vi "FolderSyncTool.vi"() -> ()   [LabVIEW 2023]
panel:
  out "Log":string
  out "file in tmp dir":path
  out "Copy Complete":bool
  in  "Dest Path":path
  in  "Source Path":path
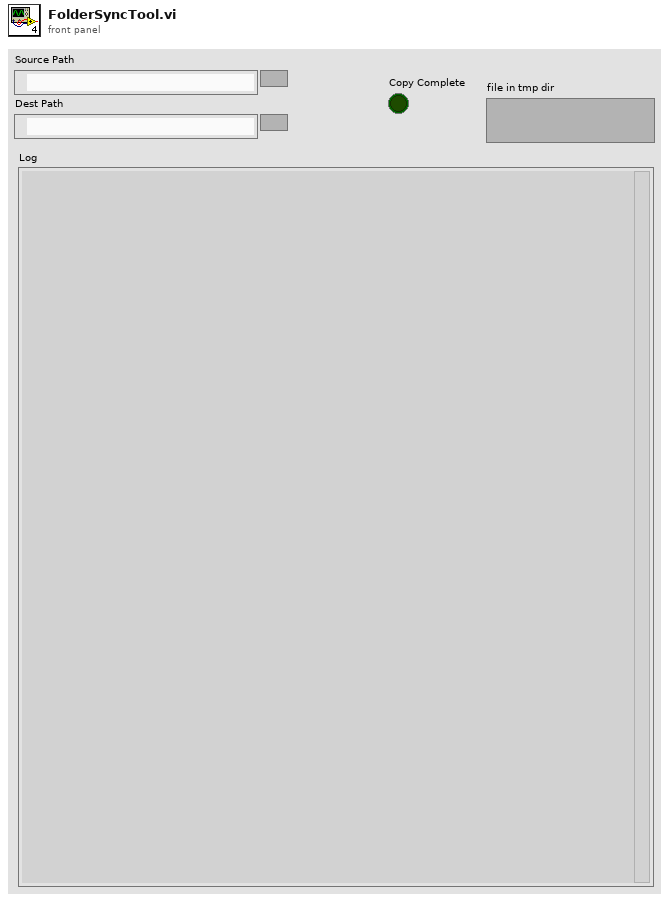
[diagram p1: front panel]
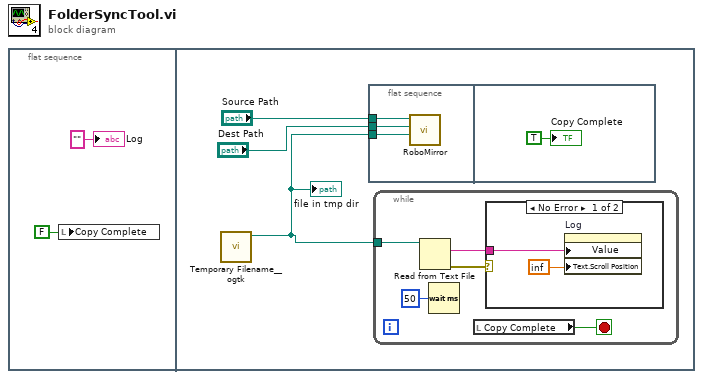
[diagram p0: block diagram]
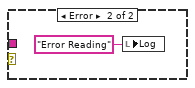
[diagram p2: hidden frame]
diagram:
  n1 = flat-sequence {
    frame #0 {
      n2 = local write "Copy Complete"(FALSE ("Copy Complete")) -> ()
      "Log" <- "" ("Log")
    }
    frame #1 {
      n3 = call <userlib>:"Temporary Filename__ogtk.vi"() -> ("file in tmp dir"=w3:path)  [unwired: 6 in, 1 out]
      "file in tmp dir" <- w3
      n4 = flat-sequence {
        tunnel: "Source Path" -> [w8]
        tunnel: "Dest Path" -> [w7]
        tunnel: w3 -> [w6]
        frame #0 {
          n5 = call "RoboMirror.vi"("Log Path"=w6, "Dest Path"=w7, "Source Path"=w8) -> ()  [unwired: 8 in, 1 out]
        }
        frame #1 {
          "Copy Complete" <- TRUE ("Copy Complete")
        }
      }
      n6 = while {
        tunnel: w3 -> [w12]
        stop <- w14 stop-if-true
        n7 = Read from Text File(file (use dialog)=w12) -> (text=w10:string, error out=w11:errorcluster)  [unwired: 3 in, 2 out]
        n8 = Wait (ms)(milliseconds to wait=u32 50) -> ()  [unwired: 1 out]
        n9 = local read "Copy Complete"() -> (w14:bool)
        n10 = case shown="No Error" w11 {
          tunnel: w10 -> [w16 _]
          frame No Error {
            n11 = property on="Log" class="Str"("Value"=w16, "Text.Scroll Position"=inf) -> ()  [unwired: 2 in, 2 out]
          }
          frame Error {
            n12 = local write "Log"("Error Reading" ("Log")) -> ()
          }
        }
      }
    }
  }
